vi "Draw Origin.vi"(6 "color (black)":u32(colorbox), 8 "frame angle (rad)":dbl, 9 "picture info":T1={"picture size"={"Width"=500, "Height"=500}, "pixels per unit"=10.0}, 10 "frame offset position":cluster{"x":dbl, "y":dbl}, 11 "picture in":picture) -> (3 "picture out":picture)   [LabVIEW 2017, in "NI_Robotics_Steering Picture.lvlib"]
uses:
  <vilib>/robotics/Utilities/Visualization/Steering Visualization/Steering Picture/NI_Robotics_Steering Picture.lvlib
  <vilib>/robotics/Utilities/Visualization/Steering Visualization/Steering Picture/Picture Info.ctl
  <vilib>/Utility/miscctls.llb/LVBoundsTypeDef.ctl
  <vilib>/Analysis/coordinate.llb/2D Cartesian Coordinate Rotation (Array).vi
  <vilib>/Analysis/NI_AALPro.lvlib
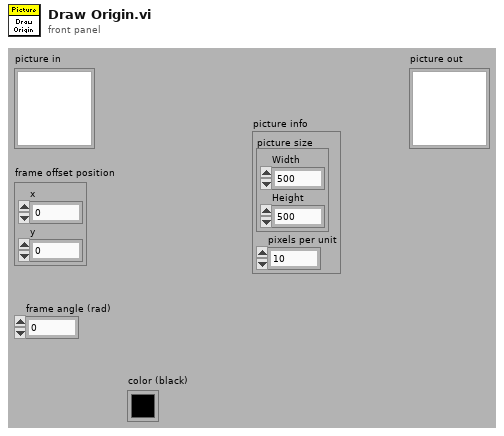
[diagram p1: front panel]
types:
  T1 = typedef "NI_Robotics_Steering Picture.lvlib/Picture Info.ctl" = cluster{"picture size":T2, "pixels per unit":dbl}
  T2 = typedef "LVBoundsTypeDef.ctl" = cluster{"Width":u32, "Height":u32}
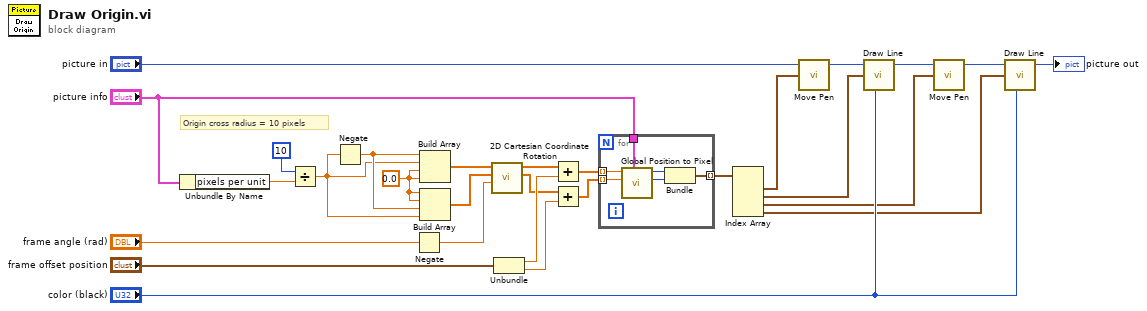
[diagram p0: block diagram]
diagram:
  w11 = 0.0 ("element")
  # "Origin cross radius = 10 pixels"
  n1 = Unbundle By Name("picture info") -> ("pixels per unit"=w21:dbl)
  n2 = Divide(x=i16 10 ("y"), y=w21) -> (x/y=w9:dbl)
  n3 = Negate(x=w9) -> (-x=w10:dbl)
  n4 = Negate(x="frame angle (rad)") -> (-x=w18:dbl)
  n5 = Build Array(w10, w9, w11, w11) -> (w7:dbl[])
  n6 = Build Array(w11, w11, w10, w9) -> (w6:dbl[])
  n7 = call-poly <vilib>:"2D Cartesian Coordinate Rotation.vi"("theta"=w18, "Y"=w6, "X"=w7) -> ("Y Out"=w2:dbl[], "X Out"=w5:dbl[])  [unwired: 6 in, 1 out]
  n8 = Unbundle("frame offset position") -> ("x"=w4:dbl, "y"=w8:dbl)
  n9 = Add(x=w5, y=w4) -> (x+y=w3:dbl[])
  n10 = Add(x=w2, y=w8) -> (x+y=w1:dbl[])
  n11 = for {
    tunnel: [w32] -> w17 mode=indexing
    tunnel: "picture info" -> [w31]
    tunnel: w3 -> [w30] mode=indexing
    tunnel: w1 -> [w29] mode=indexing
    n12 = call <vilib>:"Global Position to Pixel.vi"("picture info"=w31, "global y"=w29, "global x"=w30) -> ("pixel y"=w33:i16, "pixel x"=w34:i16)  [unwired: 7 in]
    n13 = Bundle("pixel x"=w34, "pixel y"=w33) -> (w32:cluster{"pixel x":i16, "pixel y":i16})  [unwired: 1 in]
  }
  n14 = Index Array(array=w17) -> (element #1=w16:cluster{"pixel x":i16, "pixel y":i16}, element #2=w15:cluster{"pixel x":i16, "pixel y":i16}, element #3=w14:cluster{"pixel x":i16, "pixel y":i16}, element #4=w13:cluster{"pixel x":i16, "pixel y":i16})  [unwired: 4 in]
  n15 = call <vilib>:"Move Pen.vi"("new position"=w16, "picture"="picture in") -> ("new picture"=w27:picture)  [unwired: 3 in]
  n16 = call <vilib>:"Draw Line.vi"("picture"=w27, "end point"=w15, "color(black)"="color (black)") -> ("new picture"=w26:picture)  [unwired: 6 in]
  n17 = call <vilib>:"Move Pen.vi"("new position"=w14, "picture"=w26) -> ("new picture"=w25:picture)  [unwired: 3 in]
  n18 = call <vilib>:"Draw Line.vi"("picture"=w25, "end point"=w13, "color(black)"="color (black)") -> ("new picture"=→"picture out":picture)  [unwired: 6 in]
